vi "To Waveform.vi"(8 "error in (no error)":errorcluster, 11 "Request Data in":refnum<class "Timed Data.lvclass">) -> (0 "error out":errorcluster, 1 "Success?":bool, 3 "Waveform Array":waveform(dbl)[](array[waveform]))   [LabVIEW 2020, in "Publisher.lvlib" / "Timed Data.lvclass"]
doc: "Interpret 'Data' as a Waveform Array. If impossible 'Success?' is set to FALSE\n\nThis implementation returns the Start time as t0 of the first array element."
uses:
  Timed Data.lvclass
  Timed Data.lvclass/Timed Data.ctl
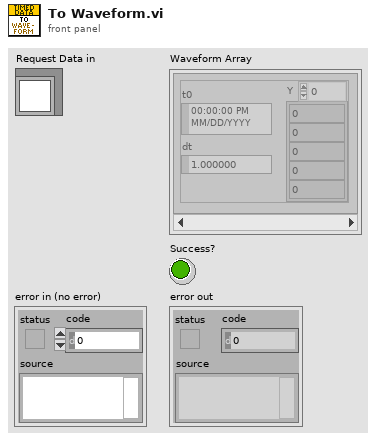
[diagram p1: front panel]
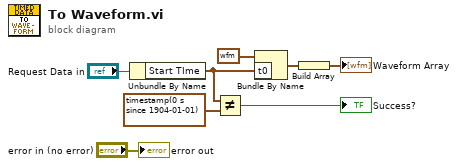
[diagram p0: block diagram]
diagram:
  n1 = Unbundle By Name("Request Data in") -> ("Start TIme"=w3:timestamp)
  n2 = Not Equal?(x=w3, y=timestamp(0 s since 1904-01-01) ("t0")) -> (x != y?=→"Success?":bool)
  n3 = Bundle By Name(cluster=waveform(dbl) {"t0"=timestamp(0 s since 1904-01-01), "dt"=1.0, "Y"=[]} ("Waveform Array"), "t0"=w3) -> (w2:waveform(dbl))
  n4 = Build Array(w2) -> (→"Waveform Array":waveform(dbl)[])
  "error out" <- "error in (no error)"
